vi "总磷总氮测量数据储存.vi"   [LabVIEW 2016, in "斯坦道总磷总氮.lvlib"]
uses:
  <vilib>/ptbypt/NI_PtbyPt.lvlib
types:
  T1 = cluster{"跨度值":dbl, "零点标准液浓度":dbl, "跨度标准液浓度":dbl, "标准液标准浓度":dbl}
  T2 = cluster{"系统时间":timestamp, "工作状态":u16, "测量模式":enum16{"待机", "连续模式", "周期模式", "定点模式", "受控模式", "手动模式"}, "告警代码":u16, "故障代码":u16, "日志代码":u16, "软件版本":u16, "F0":sgl, "F1":sgl, "F2":sgl, "F3":sgl, "T":sgl, "H":sgl, "id":u16, "flowid":u16, "量程":u16, "总磷控温温度1":sgl, "营养盐控温温度2":sgl, "ADC":sgl}
  T3 = cluster{"运行模式":enum16{"维护模式", "常规模式", "应急模式", "质控模式", "性能测试"}, "质控频次":enum16{"关闭", "每天", "星期一", "星期二", "星期三", "星期四", "星期五", "星期六", "星期日"}, "空白核查时间":u16, "跨度核查时间":u16, "测量间隔":u16}
  T4 = cluster{"因子编码":u32, "单位":u16, "标样参考值":sgl, "水样数据时间":timestamp, "水样实测值":sgl, "水样数据标识":string, "标样数据时间":timestamp, "标样实测值":sgl, "标样数据标识":string, "空白数据时间":timestamp, "空白实测值":sgl, "空白数据标识":string, "零点核查数据时间":timestamp, "零点核查实测值":sgl, "零点核查数据标识":string, "跨度核查数据时间":timestamp, "跨度核查实测值":sgl, "跨度核查数据标识":string, "加标回收数据时间":timestamp, "加标回收实测值":sgl, "加标回收数据标识":string, "平行样数据时间":timestamp, "平行样实测值":sgl, "平行样数据标识":string, "F0":sgl, "F1":sgl, "F2":sgl, "F3":sgl, "F4":sgl, "F5":sgl, "F6":sgl, "F7":sgl, "温度":sgl, "湿度":sgl, "X值":sgl, "fidrange":u16, "X1值":sgl}[]
  T5 = cluster{"总磷跨度值":dbl, "总磷零点标准液浓度":dbl, "总磷跨度标准液浓度":dbl, "总磷标准液标准浓度":dbl, "总氮跨度值":dbl, "总氮零点标准液浓度":dbl, "总氮跨度标准液浓度":dbl, "总氮标准液标准浓度":dbl, "COD跨度值":dbl, "COD零点标准液浓度":dbl, "COD跨度标准液浓度":dbl, "COD标准液标准浓度":dbl, "氨氮跨度值":dbl, "氨氮零点标准液浓度":dbl, "氨氮跨度标准液浓度":dbl, "氨氮标准液标准浓度":dbl, "磷酸盐跨度值":dbl, "磷酸盐零点标准液浓度":dbl, "磷酸盐跨度标准液浓度":dbl, "磷酸盐标准液标准浓度":dbl, "硝氮跨度值":dbl, "硝氮零点标准液浓度":dbl, "硝氮跨度标准液浓度":dbl, "硝氮标准液标准浓度":dbl, "亚硝氮跨度值":dbl, "亚硝氮零点标准液浓度":dbl, "亚硝氮跨度标准液浓度":dbl, "亚硝氮标准液标准浓度":dbl, "硫化物跨度值":dbl, "硫化物零点标准液浓度":dbl, "硫化物跨度标准液浓度":dbl, "硫化物标准液标准浓度":dbl, "硅酸盐跨度值":dbl, "硅酸盐零点标准液浓度":dbl, "硅酸盐跨度标准液浓度":dbl, "硅酸盐标准液标准浓度":dbl, "总磷零点标准液偏差":dbl, "总磷跨度标准液偏差":dbl, "总磷标准液标准偏差":dbl, "总氮零点标准液偏差":dbl, "总氮跨度标准液偏差":dbl, "总氮标准液标准偏差":dbl, "COD零点标准液偏差":dbl, "COD跨度标准液偏差":dbl, "COD标准液标准偏差":dbl, "氨氮零点标准液偏差":dbl, "氨氮跨度标准液偏差":dbl, "氨氮标准液标准偏差":dbl, "磷酸盐零点标准液偏差":dbl, "磷酸盐跨度标准液偏差":dbl, "磷酸盐标准液标准偏差":dbl, "硝氮零点标准液偏差":dbl, "硝氮跨度标准液偏差":dbl, "硝氮标准液标准偏差":dbl, "亚硝氮零点标准液偏差":dbl, "亚硝氮跨度标准液偏差":dbl, "亚硝氮标准液标准偏差":dbl, "硫化物零点标准液偏差":dbl, "硫化物跨度标准液偏差":dbl, "硫化物标准液标准偏差":dbl, "硅酸盐零点标准液偏差":dbl, "硅酸盐跨度标准液偏差":dbl, "硅酸盐标准液标准偏差":dbl, "氟化物跨度值":dbl, "氟化物零点标准液浓度":dbl, "氟化物跨度标准液浓度":dbl, "氟化物标准液标准浓度":dbl, "氟化物零点标准液偏差":dbl, "氟化物跨度标准液偏差":dbl, "氟化物标准液标准偏差":dbl, "CODMn跨度值":dbl, "CODMn零点标准液浓度":dbl, "CODMn跨度标准液浓度":dbl, "CODMn标准液标准浓度":dbl, "CODMn零点标准液偏差":dbl, "CODMn跨度标准液偏差":dbl, "CODMn标准液标准偏差":dbl}
  T6 = enum16{"水样测试", "标样核查", "跨度核查", "零点核查", "加标回收", "空白测试", "平行样"}[]
  T7 = cluster{"因子编码":u32, "单位":u16, "标样参考值":sgl, "水样数据时间":timestamp, "水样实测值":sgl, "水样数据标识":string, "标样数据时间":timestamp, "标样实测值":sgl, "标样数据标识":string, "空白数据时间":timestamp, "空白实测值":sgl, "空白数据标识":string, "零点核查数据时间":timestamp, "零点核查实测值":sgl, "零点核查数据标识":string, "跨度核查数据时间":timestamp, "跨度核查实测值":sgl, "跨度核查数据标识":string, "加标回收数据时间":timestamp, "加标回收实测值":sgl, "加标回收数据标识":string, "平行样数据时间":timestamp, "平行样实测值":sgl, "平行样数据标识":string, "F0":sgl, "F1":sgl, "F2":sgl, "F3":sgl, "F4":sgl, "F5":sgl, "F6":sgl, "F7":sgl, "温度":sgl, "湿度":sgl, "X值":sgl, "fidrange":u16, "X1值":sgl}
  T8 = typedef "斯坦道总磷总氮.lvlib/关键参数.ctl" = cluster{"测量量程":sgl, "测量检出限":sgl, "测量精度":sgl, "测量间隔":sgl, "消解温度":sgl, "消解时长":sgl, "三项式系数":sgl, "二次多项式系数":sgl, "曲线斜率":sgl, "曲线截距":sgl, "线性相关系数":sgl, "空白校准时间":timestamp, "标样校准时间":timestamp, "测量信号值":sgl, "稀释倍数":sgl, "空白标定系数":sgl, "量程系数":sgl}
  T9 = cluster{"时间标识":timestamp, "测量模式":enum16{"维护数据", "水样测试", "标样核查", "零点核查", "跨度核查", "空白测试", "平行样测试", "加标回收", "空白校准", "标样校准", "初始化（清洗）", "快捷测试"}, "数据标记表":string, "监测值":sgl, "单位":u16, "数据标识":string, "因子编码":u32, "标样参考值":sgl, "F0":sgl, "F1":sgl, "F2":sgl, "F3":sgl, "F4":sgl, "F5":sgl, "F6":sgl, "F7":sgl, "X":sgl, "温度":sgl, "湿度":sgl, "量程标识":string, "SN":string, "跨度值":sgl, "X1":sgl}
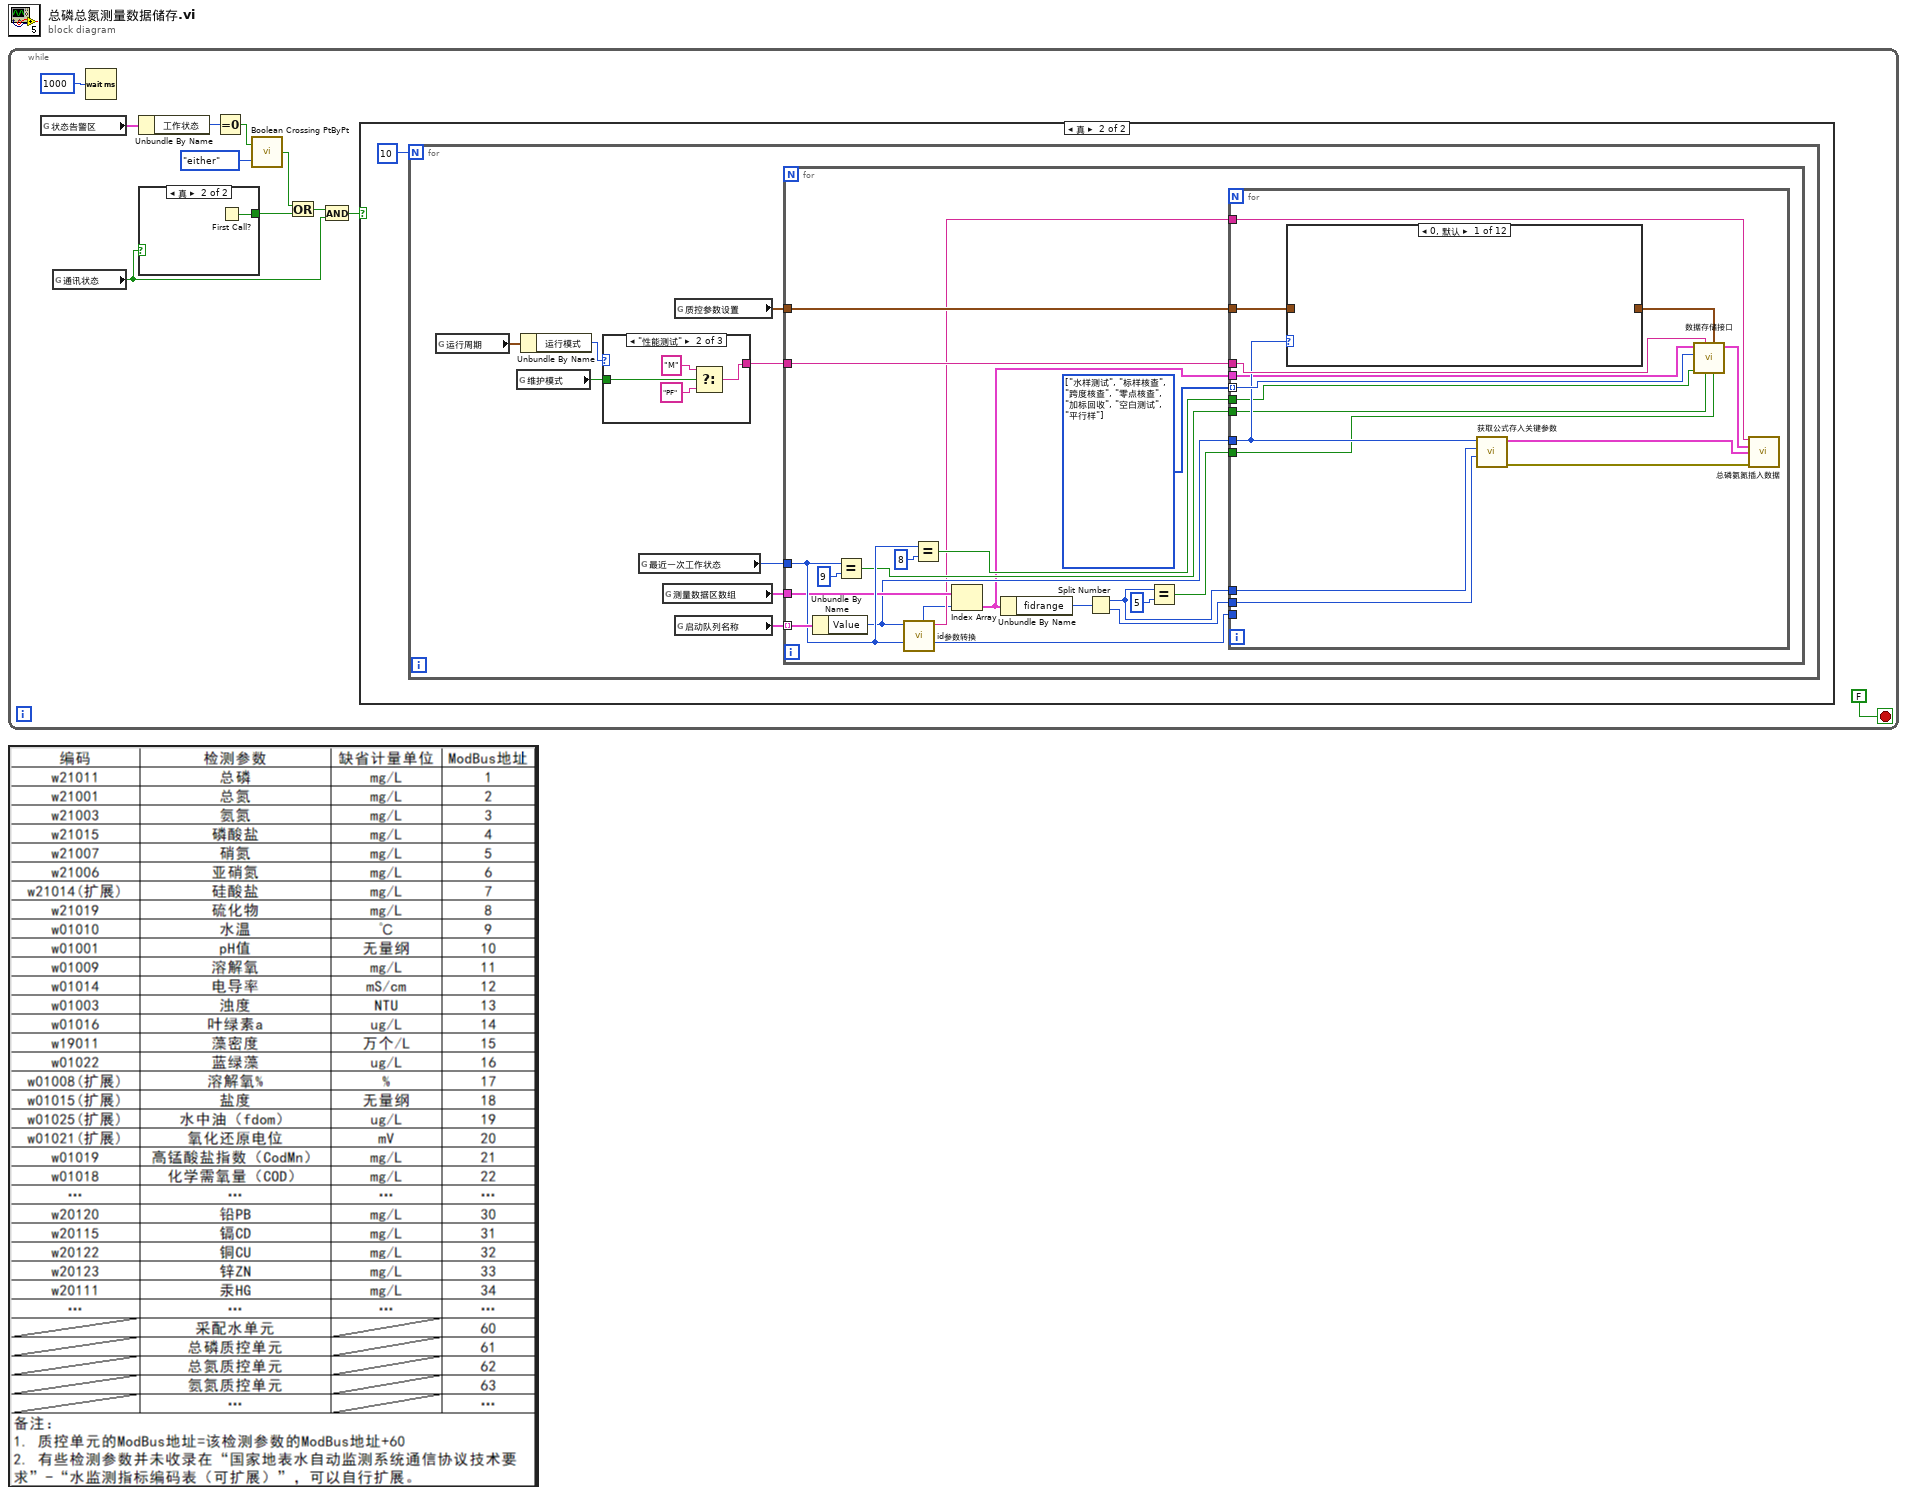
[diagram p0: block diagram]
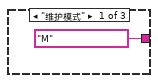
[diagram p4: hidden frame]
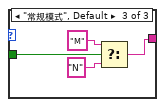
[diagram p5: hidden frame]
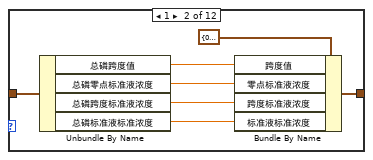
[diagram p6: hidden frame]
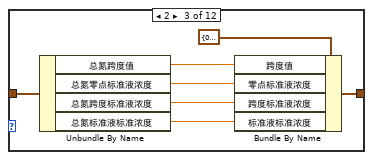
[diagram p7: hidden frame]
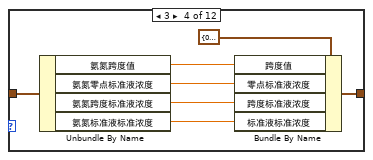
[diagram p8: hidden frame]
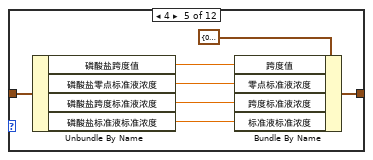
[diagram p9: hidden frame]
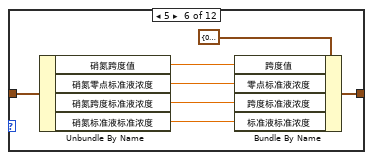
[diagram p10: hidden frame]
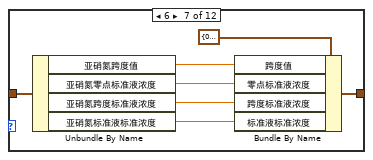
[diagram p11: hidden frame]
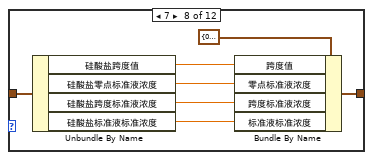
[diagram p12: hidden frame]
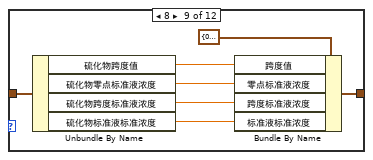
[diagram p13: hidden frame]
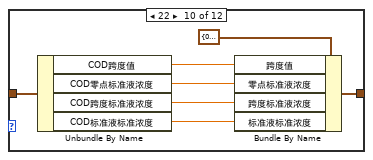
[diagram p14: hidden frame]
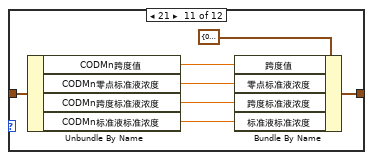
[diagram p15: hidden frame]
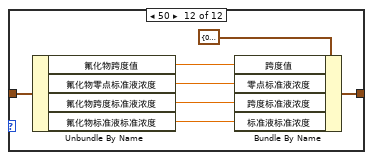
[diagram p16: hidden frame]
diagram:
  n1 = while {
    stop <- FALSE stop-if-true
    n2 = global read "VAR总磷总氮全局变量.vi" "状态告警区"() -> (w10:T2)
    n3 = global read "VAR总磷总氮全局变量.vi" "通讯状态"() -> (w3:bool)
    n4 = Wait (ms)(milliseconds to wait=u32 1000 ("等待时间（毫秒）")) -> ()  [unwired: 1 out]
    n5 = Unbundle By Name(w10) -> ("工作状态"=w8:u16)
    n6 = case shown="真" w3 {
      tunnel: [_ w12] -> w1
      frame False {
      }
      frame True {
        n7 = First Call?() -> (First Call?: T/F=w12:bool)
      }
    }
    n8 = Equal To 0?(x=w8) -> (x = 0?=w5:bool)
    n9 = call <vilib>:"Boolean Crossing PtByPt.vi"("direction"=enum16{"either", "false-true", "true-false"}."either", "input"=w5) -> ("crossing"=w6:bool)  [unwired: 1 in]
    n10 = Or(x=w6, y=w1) -> (x .or. y?=w2:bool)
    n11 = And(x=w2, y=w3) -> (x .and. y?=w4:bool)
    n12 = case shown="真" w4 {
      frame False {
      }
      frame True {
        n13 = for {
          N: 10 -> [_]
          n14 = global read "总磷总氮断电保存全局变量.vi" "运行周期"() -> (w17:T3)
          n15 = global read "总磷总氮断电保存全局变量.vi" "维护模式"() -> (w14:bool)
          n16 = Unbundle By Name(w17) -> ("运行模式"=w15:enum16{"维护模式", "常规模式", "应急模式", "质控模式", "性能测试"})
          n17 = case shown="\"性能测试\"" w15 {
            tunnel: ["M" ("数据标记表") w23 w27] -> w16
            tunnel: w14 -> [_ w24 w30]
            frame "维护模式" {
            }
            frame "性能测试" {
              n18 = Select(t="M", s=w24, f="PF") -> (s? t:f=w23:string)
            }
            frame "常规模式", Default {
              n19 = Select(t="M", s=w30, f="N") -> (s? t:f=w27:string)
            }
          }
          n20 = global read "VAR总磷总氮全局变量.vi" "最近一次工作状态"() -> (w20:u16)
          n21 = global read "VAR总磷总氮全局变量.vi" "测量数据区数组"() -> (w19:T4)
          n22 = global read "总磷总氮断电保存全局变量.vi" "质控参数设置"() -> (w18:T5)
          n23 = global read "model config var.vi" "启动队列名称"() -> (w21:cluster{"String":string, "Value":u16}[])
          n24 = for {
            tunnel: w21 -> [w46] mode=indexing
            tunnel: w20 -> [w42]
            tunnel: w19 -> [w40]
            tunnel: w18 -> [w48]
            tunnel: w16 -> [w47]
            w49 = T6 [enum."水样测试", enum."标样核查", enum."跨度核查", enum."零点核查", enum."加标回收", enum."空白测试", enum."平行样"] items=["水样测试", "标样核查", "跨度核查", "零点核查", "加标回收", "空白测试", "平行样"]
            n25 = Unbundle By Name(w46) -> ("Value"=w39:u16)
            n26 = Equal?(x=w42, y=u16 9) -> (x = y?=w41:bool)
            n27 = call "id参数转换.vi"("id"=w39) -> ("table输出"=w38:string, "数组资源索引"=w31:i32)  [unwired: 9 in]
            n28 = Equal?(x=w42, y=u16 8) -> (x = y?=w44:bool)
            n29 = Index Array(array=w40, index=w31) -> (element=w35:T7)
            n30 = Unbundle By Name(w35) -> ("fidrange"=w37:u16)
            n31 = Split Number(x=w37) -> (hi(x)=w32:u8, lo(x)=w33:u8)
            n32 = Equal?(x=w32, y=u16 5) -> (x = y?=w34:bool)
            n33 = for {
              tunnel: w49 -> [w61] mode=indexing
              tunnel: w42 -> [_]
              tunnel: w48 -> [w59]
              tunnel: w47 -> [w58]
              tunnel: w39 -> [w57]
              tunnel: w44 -> [w56]
              tunnel: w41 -> [w55]
              tunnel: w35 -> [w54]
              tunnel: w38 -> [w53]
              tunnel: w34 -> [w52]
              tunnel: w33 -> [w51]
              tunnel: w32 -> [w50]
              n34 = case shown="0, 默认" w57 {
                tunnel: w59 -> [_ w71 w78 w85 w92 w99 w106 w113 w120 w127 w134 w141]
                tunnel: [_ w69 w76 w83 w90 w97 w104 w111 w118 w125 w132 w139] -> w63
                frame 0, Default {
                }
                frame 1 {
                  n35 = Unbundle By Name(w71) -> ("总磷跨度值"=w68:dbl, "总磷零点标准液浓度"=w67:dbl, "总磷跨度标准液浓度"=w66:dbl, "总磷标准液标准浓度"=w65:dbl)
                  n36 = Bundle By Name(cluster=T1 {"跨度值"=0.0, "零点标准液浓度"=0.0, "跨度标准液浓度"=0.0, "标准液标准浓度"=0.0} ("质控参数设置"), "跨度值"=w68, "零点标准液浓度"=w67, "跨度标准液浓度"=w66, "标准液标准浓度"=w65) -> (w69:T1)
                }
                frame 2 {
                  n37 = Unbundle By Name(w78) -> ("总氮跨度值"=w75:dbl, "总氮零点标准液浓度"=w74:dbl, "总氮跨度标准液浓度"=w73:dbl, "总氮标准液标准浓度"=w72:dbl)
                  n38 = Bundle By Name(cluster=T1 {"跨度值"=0.0, "零点标准液浓度"=0.0, "跨度标准液浓度"=0.0, "标准液标准浓度"=0.0} ("质控参数设置"), "跨度值"=w75, "零点标准液浓度"=w74, "跨度标准液浓度"=w73, "标准液标准浓度"=w72) -> (w76:T1)
                }
                frame 3 {
                  n39 = Unbundle By Name(w85) -> ("氨氮跨度值"=w82:dbl, "氨氮零点标准液浓度"=w81:dbl, "氨氮跨度标准液浓度"=w80:dbl, "氨氮标准液标准浓度"=w79:dbl)
                  n40 = Bundle By Name(cluster=T1 {"跨度值"=0.0, "零点标准液浓度"=0.0, "跨度标准液浓度"=0.0, "标准液标准浓度"=0.0} ("质控参数设置"), "跨度值"=w82, "零点标准液浓度"=w81, "跨度标准液浓度"=w80, "标准液标准浓度"=w79) -> (w83:T1)
                }
                frame 4 {
                  n41 = Unbundle By Name(w92) -> ("磷酸盐跨度值"=w89:dbl, "磷酸盐零点标准液浓度"=w88:dbl, "磷酸盐跨度标准液浓度"=w87:dbl, "磷酸盐标准液标准浓度"=w86:dbl)
                  n42 = Bundle By Name(cluster=T1 {"跨度值"=0.0, "零点标准液浓度"=0.0, "跨度标准液浓度"=0.0, "标准液标准浓度"=0.0} ("质控参数设置"), "跨度值"=w89, "零点标准液浓度"=w88, "跨度标准液浓度"=w87, "标准液标准浓度"=w86) -> (w90:T1)
                }
                frame 5 {
                  n43 = Unbundle By Name(w99) -> ("硝氮跨度值"=w96:dbl, "硝氮零点标准液浓度"=w95:dbl, "硝氮跨度标准液浓度"=w94:dbl, "硝氮标准液标准浓度"=w93:dbl)
                  n44 = Bundle By Name(cluster=T1 {"跨度值"=0.0, "零点标准液浓度"=0.0, "跨度标准液浓度"=0.0, "标准液标准浓度"=0.0} ("质控参数设置"), "跨度值"=w96, "零点标准液浓度"=w95, "跨度标准液浓度"=w94, "标准液标准浓度"=w93) -> (w97:T1)
                }
                frame 6 {
                  n45 = Unbundle By Name(w106) -> ("亚硝氮跨度值"=w103:dbl, "亚硝氮零点标准液浓度"=w102:dbl, "亚硝氮跨度标准液浓度"=w101:dbl, "亚硝氮标准液标准浓度"=w100:dbl)
                  n46 = Bundle By Name(cluster=T1 {"跨度值"=0.0, "零点标准液浓度"=0.0, "跨度标准液浓度"=0.0, "标准液标准浓度"=0.0} ("质控参数设置"), "跨度值"=w103, "零点标准液浓度"=w102, "跨度标准液浓度"=w101, "标准液标准浓度"=w100) -> (w104:T1)
                }
                frame 7 {
                  n47 = Unbundle By Name(w113) -> ("硅酸盐跨度值"=w110:dbl, "硅酸盐零点标准液浓度"=w109:dbl, "硅酸盐跨度标准液浓度"=w108:dbl, "硅酸盐标准液标准浓度"=w107:dbl)
                  n48 = Bundle By Name(cluster=T1 {"跨度值"=0.0, "零点标准液浓度"=0.0, "跨度标准液浓度"=0.0, "标准液标准浓度"=0.0} ("质控参数设置"), "跨度值"=w110, "零点标准液浓度"=w109, "跨度标准液浓度"=w108, "标准液标准浓度"=w107) -> (w111:T1)
                }
                frame 8 {
                  n49 = Unbundle By Name(w120) -> ("硫化物跨度值"=w117:dbl, "硫化物零点标准液浓度"=w116:dbl, "硫化物跨度标准液浓度"=w115:dbl, "硫化物标准液标准浓度"=w114:dbl)
                  n50 = Bundle By Name(cluster=T1 {"跨度值"=0.0, "零点标准液浓度"=0.0, "跨度标准液浓度"=0.0, "标准液标准浓度"=0.0} ("质控参数设置"), "跨度值"=w117, "零点标准液浓度"=w116, "跨度标准液浓度"=w115, "标准液标准浓度"=w114) -> (w118:T1)
                }
                frame 22 {
                  n51 = Unbundle By Name(w127) -> ("COD跨度值"=w124:dbl, "COD零点标准液浓度"=w123:dbl, "COD跨度标准液浓度"=w122:dbl, "COD标准液标准浓度"=w121:dbl)
                  n52 = Bundle By Name(cluster=T1 {"跨度值"=0.0, "零点标准液浓度"=0.0, "跨度标准液浓度"=0.0, "标准液标准浓度"=0.0} ("质控参数设置"), "跨度值"=w124, "零点标准液浓度"=w123, "跨度标准液浓度"=w122, "标准液标准浓度"=w121) -> (w125:T1)
                }
                frame 21 {
                  n53 = Unbundle By Name(w134) -> ("CODMn跨度值"=w131:dbl, "CODMn零点标准液浓度"=w130:dbl, "CODMn跨度标准液浓度"=w129:dbl, "CODMn标准液标准浓度"=w128:dbl)
                  n54 = Bundle By Name(cluster=T1 {"跨度值"=0.0, "零点标准液浓度"=0.0, "跨度标准液浓度"=0.0, "标准液标准浓度"=0.0} ("质控参数设置"), "跨度值"=w131, "零点标准液浓度"=w130, "跨度标准液浓度"=w129, "标准液标准浓度"=w128) -> (w132:T1)
                }
                frame 50 {
                  n55 = Unbundle By Name(w141) -> ("氟化物跨度值"=w138:dbl, "氟化物零点标准液浓度"=w137:dbl, "氟化物跨度标准液浓度"=w136:dbl, "氟化物标准液标准浓度"=w135:dbl)
                  n56 = Bundle By Name(cluster=T1 {"跨度值"=0.0, "零点标准液浓度"=0.0, "跨度标准液浓度"=0.0, "标准液标准浓度"=0.0} ("质控参数设置"), "跨度值"=w138, "零点标准液浓度"=w137, "跨度标准液浓度"=w136, "标准液标准浓度"=w135) -> (w139:T1)
                }
              }
              n57 = call "获取公式存入关键参数.vi"("量程"=w51, "flowid"=w50, "id"=w57) -> ("error out"=w62:errorcluster, "关键参数"=w60:T8)  [unwired: 7 in]
              n58 = call "数据存储接口.vi"("快捷测试？"=w52, "质控参数设置"=w63, "标样校准？"=w55, "数据标记表"=w58, "空白校准？"=w56, "数据存储模式"=w61, "测量数据区"=w54) -> ("data输出"=w64:T9)  [unwired: 4 in]
              n59 = call "总磷氨氮插入数据.vi"("table"=w53, "data"=w64, "关键参数"=w60, "error in (no error)"=w62) -> ()  [unwired: 11 in, 1 out]
            }
          }
        }
      }
    }
  }
